vi "GenerateChangedLVFilesPath.vi"(6 "GUI Mode? {F)":bool, 8 "error in (no error)":errorcluster, 11 "Workspace Path":path=path "E:/sw-deps-monitor") -> (0 "error out":errorcluster)   [LabVIEW 2019, in "Hawkeye.lvlib"]
uses:
  Hawkeye.lvlib
  ead0c1dc-4abe-4fdf-93af-0a2c3e7fff4b.vi
  <vilib>/Wiresmith Technology/G CLI/CLI Class/CLI.lvclass
panel:
  in  "Tab Control":enum32{"GUI Mode", "CLI Mode"}(tab)=enum."CLI Mode"
  out "Args":string[](array[string])=["E:\\sw-deps-monitor"]
  # "When in GUI Mode, the controls will be used, \nin CLI Mode the Args will be used"
  # "Command to run the VI from terminal\n\ng-cli -v --lv-ver 2023 --arch 32 \"E:\\sw-deps-monitor\\CICD\\CheckModifiedVIs\\GenerateChangedLibrariesList.vi\" -- \"E:\\sw-deps-monitor\""
  # "Workspace Path"
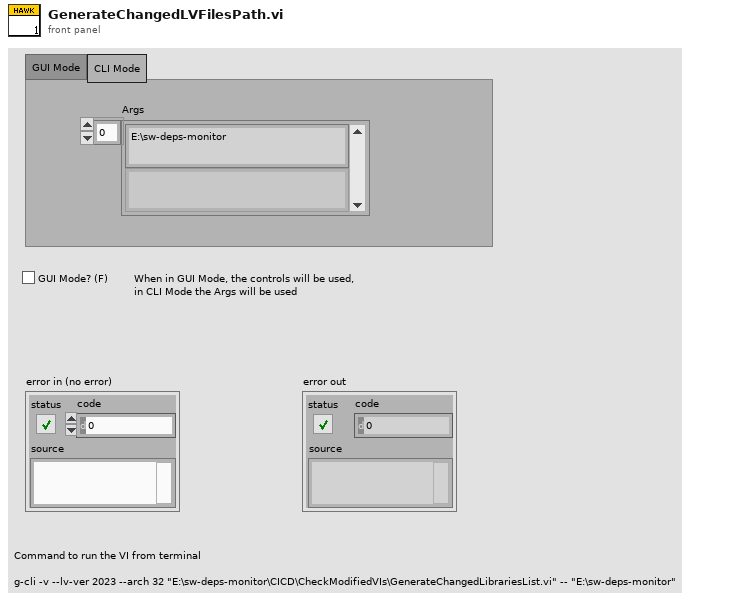
[diagram p1: front panel]
types:
  T1 = enum16{"open", "replace", "create", "open or create", "replace or create", "replace or create with confirmation"}
  T2 = typedef "Hawkeye.lvlib/HawkeyePathConfigs.ctl" = cluster{"GlobalIncludePaths":path[], "GlobalExcludePaths":path[], "BuildSpecsIncludePaths":path[], "ActualDepsIncludePaths":path[], "WorkspacePath":path, "SourceFolderPaths":path[], "ChangedFilesLogpaths":map{string, path}, "CacheRecreateDuration":dbl}
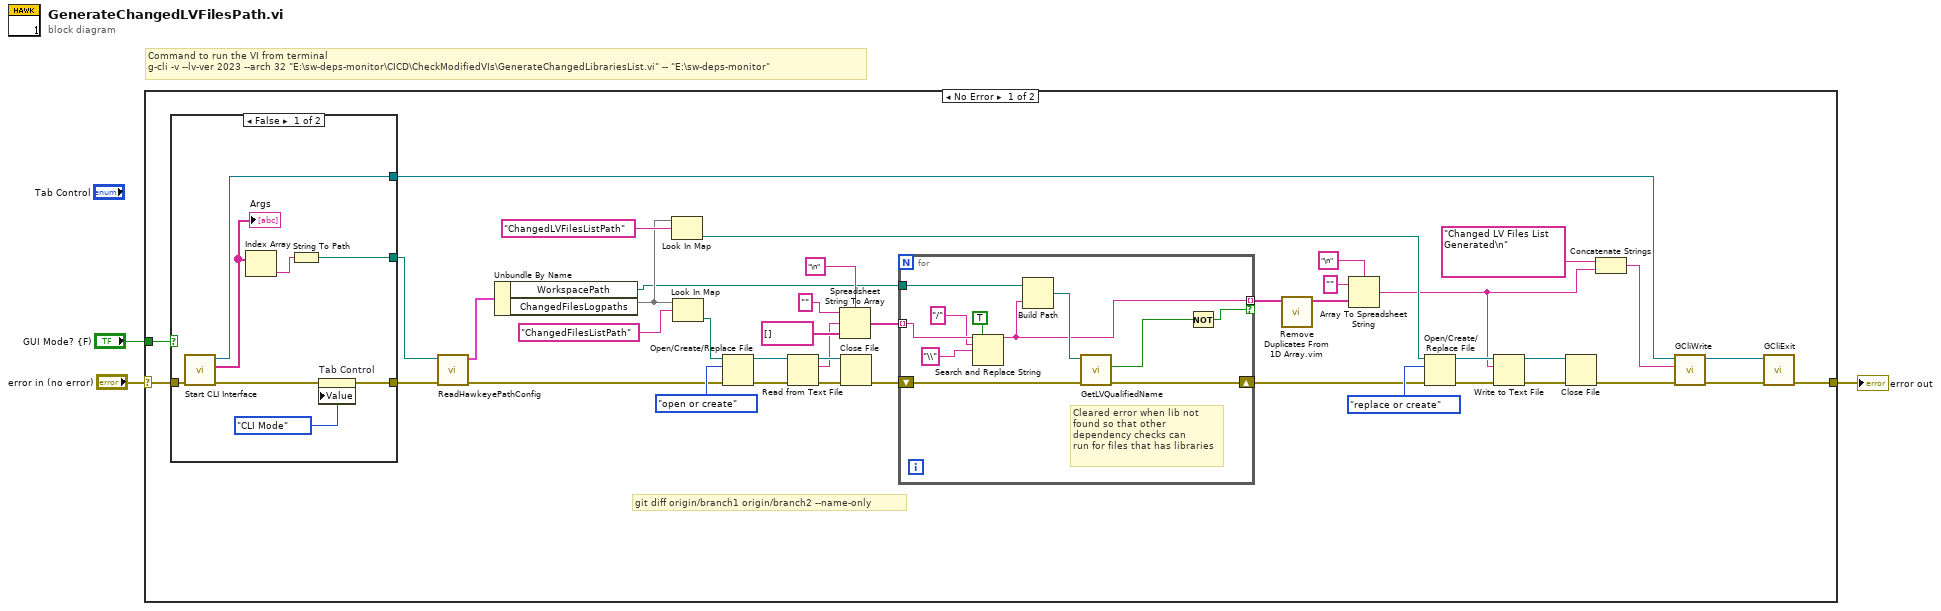
[diagram p0: block diagram]
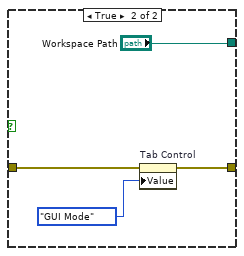
[diagram p2: hidden frame]
diagram:
  # "Command to run the VI from terminal\ng-cli -v --lv-ver 2023 --arch 32 \"E:\\sw-deps-monitor\\CICD\\CheckModifiedVIs\\GenerateChangedLibrariesList.vi\" -- \"E:\\sw-deps-monitor\""
  n1 = case shown="No Error" "error in (no error)" {
    selector: "error in (no error)" -> [w43 w68]
    tunnel: "GUI Mode? {F)" -> [w44 _]
    tunnel: [w39 w68] -> w1
    frame No Error {
      # "git diff origin/branch1 origin/branch2 --name-only"
      n2 = case shown="False" w44 {
        tunnel: [w62 "Workspace Path"] -> w36
        tunnel: w43 -> [w61 w66]
        tunnel: [w59 w64] -> w35
        tunnel: [w60 _] -> w41
        frame False {
          n3 = call <vilib>:"Start CLI Interface.vi"("error in (no error)"=w61) -> ("error out"=w57:errorcluster, "Custom Parameters"=w56:string[], "CLI out"=w60:refnum<class "CLI.lvclass">)  [unwired: 7 in, 1 out]
          "Args" <- w56
          n4 = Index Array(array=w56) -> (element=w63:string)  [unwired: 1 in]
          n5 = String To Path(string=w63) -> (path=w62:path)
          n6 = property on="Tab Control" class="TabCtl (strict)"(error in=w57, "Value"=enum32{"GUI Mode", "CLI Mode"}."CLI Mode" ("Tab Control")) -> (error out=w59:errorcluster)  [unwired: 1 in, 1 out]
        }
        frame True {
          n7 = property on="Tab Control" class="TabCtl (strict)"(error in=w66, "Value"=enum32{"GUI Mode", "CLI Mode"}."GUI Mode" ("Tab Control")) -> (error out=w64:errorcluster)  [unwired: 1 in, 1 out]
        }
      }
      n8 = call "ReadHawkeyePathConfig.vi"("error in (no error)"=w35, "Workspace Path"=w36) -> ("error out"=w24:errorcluster, "Hawkeye Path Config Out"=w34:T2)  [unwired: 8 in]
      n9 = Unbundle By Name(w34) -> ("WorkspacePath"=w14:path, "ChangedFilesLogpaths"=w22:map{string, path})
      n10 = Look In Map(map=w22, key="ChangedLVFilesListPath") -> (value=w21:path)  [unwired: 1 in, 1 out]
      n11 = Look In Map(map=w22, key="ChangedFilesListPath") -> (value=w32:path)  [unwired: 1 in, 1 out]
      n12 = Open/Create/Replace File(file path (use dialog)=w32, error in=w24, operation (0:open)=T1."open or create") -> (refnum out=w31:refnum<file>, error out=w30:errorcluster)  [unwired: 3 in, 1 out]
      n13 = Read from Text File(file (use dialog)=w31, error in=w30) -> (refnum out=w29:refnum<file>, text=w26:string, error out=w28:errorcluster)  [unwired: 2 in, 1 out]
      n14 = Spreadsheet String To Array(delimiter (Tab)="\n", format string="", spreadsheet string=w26, array type (2D Dbl)=string[] []) -> (array=w15:string[])
      n15 = Close File(refnum=w29, error in=w28) -> (error out=w13:errorcluster)  [unwired: 1 out]
      n16 = for {
        tunnel: w15 -> [w54] mode=indexing
        tunnel: w14 -> [w55]
        tunnel: [w47] -> w6 mode=indexing if=w50
        shift-right: [w45] -> w10
        shift-left: w13 -> [w48]
        # "Cleared error when lib not\nfound so that other\ndependency checks can\nrun for files that has libraries"
        n17 = Search and Replace String(replace all?=TRUE ("replace all? (F)"), input string=w54, search string="/", replace string="\\" ("replace string (\"\")")) -> (result string=w47:string)  [unwired: 4 in, 3 out]
        n18 = Build Path(base path=w55, name or relative path=w47) -> (appended path=w49:path)
        n19 = call "GetLVQualifiedName.vi"("error in (no error)"=w48, "LV File Path"=w49) -> ("error out"=w45:errorcluster, "Non LabVIEW File?"=w46:bool)  [unwired: 7 in, 1 out]
        n20 = Not(x=w46) -> (.not. x?=w50:bool)
      }
      n21 = call "Remove Duplicates From 1D Array.vim"("array"=w6) -> ("array with duplicates removed"=w5:string[])  [unwired: 10 in]
      n22 = Array To Spreadsheet String(delimiter (Tab)="\n", array=w5, 3:"" ("format string")) -> (spreadsheet string=w9:string)
      n23 = Open/Create/Replace File(file path (use dialog)=w21, error in=w10, operation (0:open)=T1."replace or create") -> (refnum out=w18:refnum<file>, error out=w19:errorcluster)  [unwired: 3 in, 1 out]
      n24 = Write to Text File(file (use dialog)=w18, text=w9, error in=w19) -> (refnum out=w16:refnum<file>, error out=w17:errorcluster)  [unwired: 1 in, 1 out]
      n25 = Close File(refnum=w16, error in=w17) -> (error out=w8:errorcluster)  [unwired: 1 out]
      n26 = Concatenate Strings("Changed LV Files List Generated\n" ("Text to Write"), w9) -> (w4:string)
      n27 = call "GCliWrite.vi"("error in (no error)"=w8, "Text to Write"=w4, "CLI in"=w41) -> ("error out"=w40:errorcluster, "CLI out"=w38:refnum<class "CLI.lvclass">)  [unwired: 7 in]
      n28 = call "GCliExit.vi"("error in (no error)"=w40, "CLI in"=w38) -> ("error out"=w39:errorcluster)  [unwired: 9 in]
    }
    frame Error {
    }
  }
  "error out" <- w1
